vi "ReadTempAndUpdateFPGA.vi"(8 "error in (no error)":errorcluster, 9 "Sensors":T1, 10 "TempThreshold":dbl=150.0, 11 "FPGA VI Reference":T2) -> (0 "error out":errorcluster)   [LabVIEW 2019]
uses:
  FPGA VI Ref.ctl
  <vilib>/Utility/error.llb/Error Cluster From Error Code.vi
  <vilib>/rvi/errors/niLvFpgaAdjustHostInterfaceError.vi
  <vilib>/rvi/interface/nirviReadWriteControl/nirviReadWriteControl.xnode
  <vilib>/rvi/interface/Simulation/niFpgaSimulationCallBeginRW.vi
  NiFpgaLv.dll
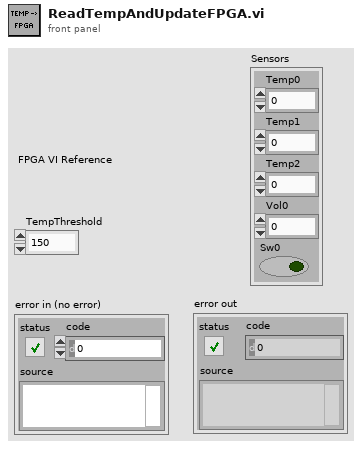
[diagram p1: front panel]
types:
  T1 = cluster{"Temp0":dbl, "Temp1":dbl, "Temp2":dbl, "Vol0":dbl, "Sw0":bool}
  T2 = typedef "FPGA VI Ref.ctl" = refnum<k20>
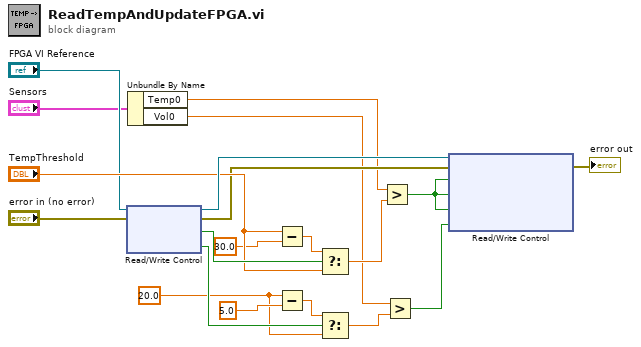
[diagram p0: block diagram]
diagram:
  w4 = 20.0 ("y")
  n1 = xnode "Read/Write Control"("FPGA VI Reference In"="FPGA VI Reference", "error in"="error in (no error)") -> ("FPGA VI Reference Out"=w18:T2, "error out"=w11:errorcluster, "Löyly LED"=w17:bool, "Aromi LED"=w7:bool)
  n2 = Unbundle By Name("Sensors") -> ("Temp0"=w10:dbl, "Vol0"=w6:dbl)
  n3 = Subtract(x="TempThreshold", y=30.0) -> (x-y=w15:dbl)
  n4 = Subtract(x=w4, y=5.0) -> (x-y=w8:dbl)
  n5 = Select(t=w15, s=w17, f="TempThreshold") -> (s? t:f=w16:dbl)
  n6 = Select(t=w8, s=w7, f=w4) -> (s? t:f=w5:dbl)
  n7 = Greater?(x=w10, y=w16) -> (0:w3:bool)
  n8 = Greater?(x=w6, y=w5) -> (0:w2:bool)
  n9 = xnode "Read/Write Control"("FPGA VI Reference In"=w18, "error in"=w11, "Aromi Pump Enable"=w3, "Löyly Valve Enable"=w3, "Löyly LED"=w3, "Aromi LED"=w2) -> ("error out"=→"error out":errorcluster)  [unwired: 1 out]
